vi "Numeric Control - Silver Table.vi"() -> ()   [LabVIEW 2012, in "TableSupportLib.lvlib"]
doc: "Sample numeric display item."
uses:
  TableSupportLib.lvlib
  <vilib>/NI Veristand/Display Template Support/Display Template Support.llb/cluster_Screen Item Settings.ctl
  <vilib>/NI Veristand/Display Template Support/Display Template Support.llb/cluster_Graph Scale Settings.ctl
  <vilib>/NI Veristand/Display Template Support/Display Template Support.llb/cluster_Graph Plot Settings.ctl
  NationalInstruments.VeriStand.SystemStorage
  <vilib>/NI Veristand/Display Template Support/Display Template Support.llb/enum_Display Template Handler Minimal To Widget Msg.ctl
  <vilib>/NI Veristand/Display Template Support/Display Template Support.llb/enum_Display Template Handler Minimal To Workspace.ctl
  SubVIs/Table_StateControl.ctl
  SubVIs/Table_StateInformation.ctl
  SubVIs/Table_ChannelInfoCluster.ctl
  SubVIs/Table_SortArraySettings.ctl
  SubVIs/Table_ListboxSettings.ctl
  <vilib>/NI Veristand/Display Template Support/Display Template Support.llb/sub_Display Template Handler Custom.vi
  <vilib>/NI Veristand/Execution/Workspace/NI VeriStand - Set Single Channel Value.vi
  SubVIs/Table_Globals.vi
  <vilib>/NI Veristand/Execution/Workspace/NI_VS Workspace ExecutionAPI.lvlib
panel:
  in  "Value":dbl
  in  "Listbox":i32(listbox)
  in  "NIVS.Gateway IP Address":string
  in  "NIVS.System Definition Root":refnum<k24>
  in  "Item.Data":T1
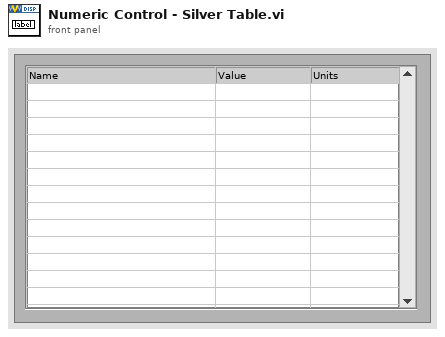
[diagram p1: front panel]
types:
  T1 = typedef "cluster_Screen Item Settings.ctl" = cluster{"Template VI":string, "Position X":i32, "Position Y":i32, "Custom":string, "Show Title Bar":bool, "ID":i32, "Always On Top":bool, "Allow Resize":bool, "Allow Minimize":bool, "Allow Close":bool, "Size to Screen":bool, "Screen.ID":i32, "State":enum16{"Normal", "New"}, "Title":string, "Window Bounds":cluster{"[0]":i16, "[1]":i16, "[2]":i16, "[3]":i16}, "Channel Ref":u64, "Unit":string, "Default Units?":bool, "Flash Limit?":bool, "Color 1":u32, "Color 2":u32, "Color 3":u32, "Color 4":u32, "Bck Color":u32, "Fore Color":u32, "Limit 1":dbl, "Limit 2":dbl, "Limit 3":dbl, "Limit 4":dbl, "Limit Mode 1":i32, "Limit Mode 2":i32, "Limit Mode 3":i32, "Limit Mode 4":i32, "Scale Precision":i32, "Scale Min":dbl, "Scale Max":dbl, "Format":i32, "Precision":i32, "Background Type":i32, "IDs":i32[], "Units":string[], "Labels":string[], "Scale Factor":dbl, "Scale Offset":dbl, "YScale Index":u32[], "XScale":T2, "YScales":T2[], "Plots":T3[], "Update Period":dbl, "History Length":dbl, "My.Ref":refnum<vi>, "Is Control?":bool, "Channel Paths":string[], "Custom Data":variant}
  T2 = typedef "cluster_Graph Scale Settings.ctl" = cluster{"Format":u8, "Precision":u8, "Fit":u8, "Label":string, "Use Default Label":bool, "Label Visible":bool, "Min":dbl, "Max":dbl}
  T3 = typedef "cluster_Graph Plot Settings.ctl" = cluster{"Bar Style":u8, "Fill To":i16, "Fill/PtColor":u32, "Line Style":u8, "Line Width":u8, "Color":u32, "Interp":u8, "Point Style":u8}
  T4 = typedef "TableSupportLib.lvlib/Table_StateControl.ctl" = enum16{"Init", "Run"}
  T5 = typedef "enum_Display Template Handler Minimal To Workspace.ctl" = cluster{"Operation":enum16{"SetCustomData", "DeleteItem"}, "Data":variant}
  T6 = typedef "enum_Display Template Handler Minimal To Widget Msg.ctl" = enum16{"Stop", "LaunchConfigDialog"}
  T7 = typedef "NI_VS Workspace ExecutionAPI.lvlib/WorkspaceAPI.ctl" = refnum<k24>
  T8 = typedef "TableSupportLib.lvlib/Table_StateInformation.ctl" = cluster{"Channel Selection":T9[], "Widths":dbl[], "Sort Info":T10, "Listbox Settings":T11}
  T9 = typedef "TableSupportLib.lvlib/Table_ChannelInfoCluster.ctl" = cluster{"NodePath":string, "Name":string, "Units":string, "Enabled":bool}
  T10 = typedef "TableSupportLib.lvlib/Table_SortArraySettings.ctl" = cluster{"Order":enum16{"ascending", "descending"}, "Column":i32}
  T11 = typedef "TableSupportLib.lvlib/Table_ListboxSettings.ctl" = cluster{"Font":u32, "Bold":bool, "Poll Rate":u32, "Enable Limits":bool, "Path":path}
  T12 = typedef "lveventtype.ctl" = enum32{"Null", "Timeout", "Annotation Menu Selection", "Annotation Menu Selection?", "App Instance Close", "App Instance Close?", "Autoscale Range Change", "Cell Edit", "Cell Edit?", "Cursor Grab", "Cursor Grab?", "Cursor Menu Selection", "Cursor Menu Selection?", "Cursor Move", "Cursor Release", "Data Change", "Direction Change", "Display State Change", "Drag Ended", "Drag Enter", "Drag Leave", "Drag Over", "Drag Source Update", "Drag Starting", "Drag Starting?", "Drop", "Exec State Change", "Key Down", "Key Down?", "Key Repeat", "Key Repeat?", "Key Up", "Listbox Double Click", "Menu Activation?", "Menu Selection (App)", "Menu Selection? (App)", "Menu Selection (User)", "Mouse Down", "Mouse Down?", "Mouse Enter", "Mouse Leave", "Mouse Move", "Mouse Up", "NI Security User Change (App)", "Pane Size", "Panel Close", "Panel Close?", "Panel Resize", "Plot Attribute Change", "Scale Range Change", "Shortcut Menu Activation?", "Shortcut Menu Selection (App)", "Shortcut Menu Selection? (App)", "Shortcut Menu Selection (User)", "Tree Double Click", "Tree Drag", "Tree Drag?", "Tree Drop", "Tree Drop?", "Tree Item Close", "Tree Item Close?", "Tree Item Open", "Tree Item Open?", "Value Change"}
  T13 = typedef "LVPoint32TypeDef.ctl" = cluster{"Horizontal":i32, "Vertical":i32}
  T14 = typedef "LVRowAndColumnTypeDef.ctl" = cluster{"Row":i32, "Column":i32}
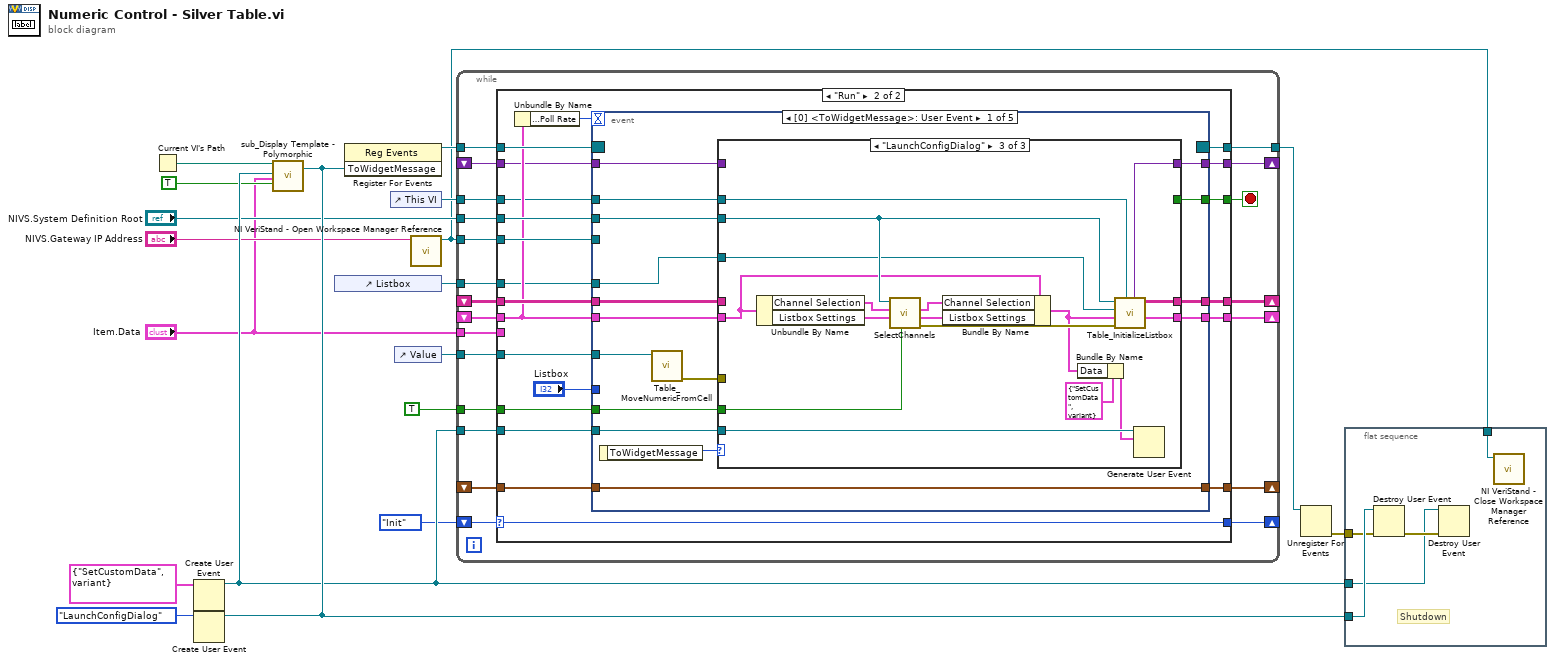
[diagram p0: block diagram]
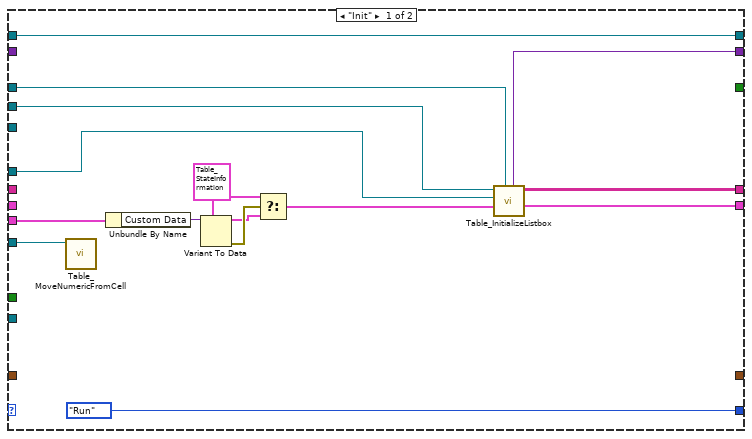
[diagram p2: hidden frame]
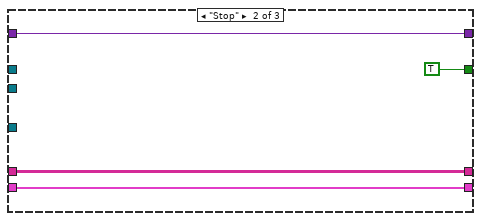
[diagram p4: hidden frame]
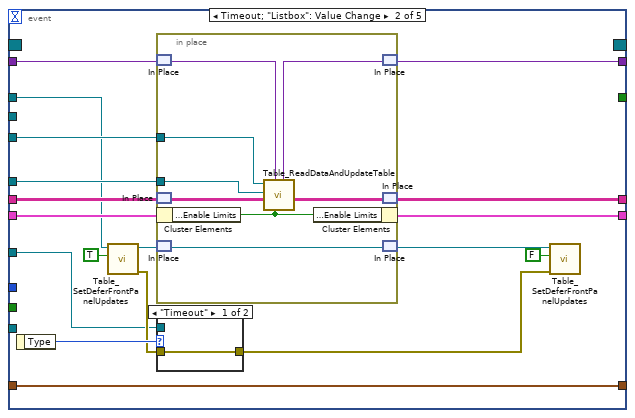
[diagram p5: hidden frame]
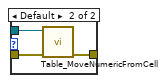
[diagram p6: hidden frame]
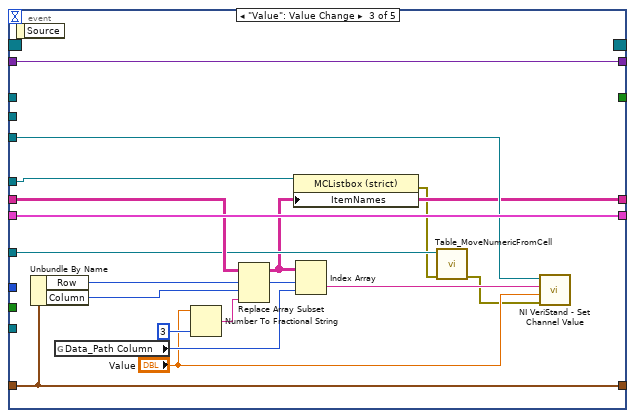
[diagram p7: hidden frame]
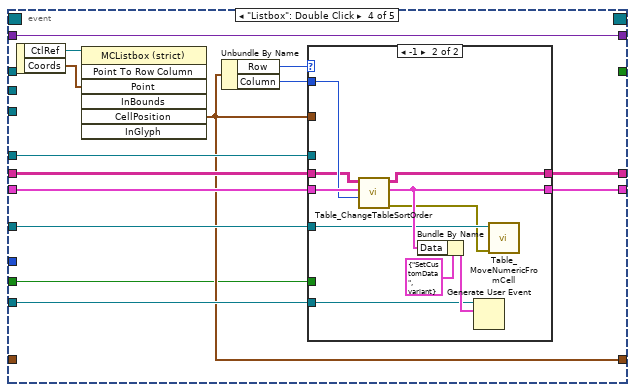
[diagram p8: hidden frame]
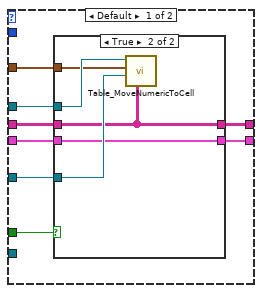
[diagram p9: hidden frame]
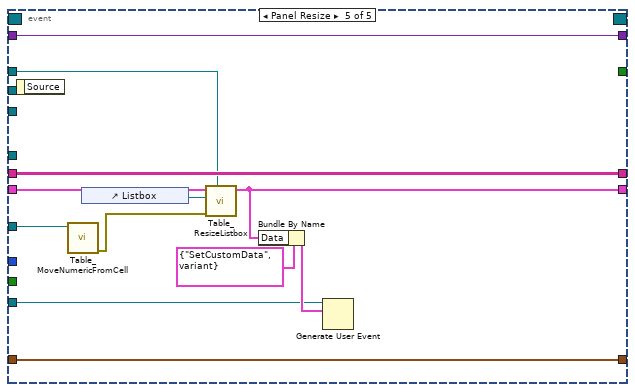
[diagram p11: hidden frame]
diagram:
  n1 = Current VI's Path() -> (path=w12:path)
  n2 = Create User Event(user event datatype=T5 {"Operation"=enum."SetCustomData", "Data"=variant} ("Data")) -> (user event=w11:refnum<user-event>)  [unwired: 1 in, 1 out]
  n3 = Create User Event(user event datatype=enum_Display_Template_Handler_Minimal_To_Widget_Msg."LaunchConfigDialog" ("ToWidgetMessage")) -> (user event=w14:refnum<user-event>)  [unwired: 1 in, 1 out]
  n4 = call-poly <vilib>:"sub_Display Template - Polymorphic.vi"("Parent.Path"=w12, "ToWidgetEvent"=w14, "ToWorkspace"=w11, "Item.Data"="Item.Data", "Resizable"=TRUE) -> ()  [unwired: 1 in, 14 out]
  n5 = control-ref of="Listbox"() -> (w4:refnum<vi>)
  n6 = register-events(w14) -> (reference out=w17:refnum<event-registration>)  [unwired: 2 in, 1 out]
  n7 = control-ref of="This VI"() -> (w5:refnum<vi>)
  n8 = control-ref of="Value"() -> (w3:refnum<vi>)
  n9 = call <vilib>:"NI VeriStand - Open Workspace Manager Reference.vi"("Gateway IP Address (\"\": localhost)"="NIVS.Gateway IP Address") -> ("WorkspaceManager"=w1:T7)  [unwired: 9 in, 1 out]
  n10 = while {
    tunnel: w17 -> [w39]
    tunnel: [w37] -> w16
    tunnel: w11 -> [w36]
    tunnel: "NIVS.System Definition Root" -> [w35]
    shift-right: [w32] -> _
    shift-left: _ -> [w34]
    tunnel: w1 -> [w33]
    shift-right: [w31] -> _
    shift-left: _ -> [w30]
    shift-right: [w28] -> _
    shift-left: Table_StateControl."Init" -> [w29]
    tunnel: "Item.Data" -> [w27]
    shift-right: [w26] -> _
    shift-left: _ -> [w25]
    tunnel: w5 -> [w24]
    tunnel: w4 -> [w23]
    tunnel: w3 -> [w22]
    shift-right: [w21] -> _
    shift-left: _ -> [w20]
    tunnel: TRUE ("Controls Only?") -> [w19]
    stop <- w38 stop-if-true
    n11 = case shown="\"Run\"" w29 {
      selector: w29 -> [_ w66]
      tunnel: w39 -> [w54 w75]
      tunnel: [_ w74] -> w38
      tunnel: [w54 w73] -> w37
      tunnel: w36 -> [_ w72]
      tunnel: w35 -> [w52 w71]
      tunnel: w34 -> [_ w65]
      tunnel: w33 -> [_ w70]
      tunnel: [w51 w69] -> w32
      tunnel: [w50 w68] -> w31
      tunnel: w30 -> [_ w67]
      tunnel: [Table_StateControl."Run" w66] -> w28
      tunnel: w27 -> [w48 _]
      tunnel: [w43 w63] -> w26
      tunnel: w25 -> [_ w62]
      tunnel: w24 -> [w42 w61]
      tunnel: w23 -> [w41 w59]
      tunnel: w22 -> [w40 w58]
      tunnel: [_ w57] -> w21
      tunnel: w20 -> [_ w56]
      tunnel: w19 -> [_ w55]
      frame "Init" {
        w46 = T8 {"Channel Selection"=[], "Widths"=[], "Sort Info"={"Order"=enum."ascending", "Column"=0}, "Listbox Settings"={"Font"=13, "Bold"=FALSE, "Poll Rate"=200, "Enable Limits"=FALSE, "Path"=path ""}}
        n12 = call "Table_MoveNumericFromCell.vi"("Digital in"=w40) -> ()  [unwired: 10 in, 1 out]
        n13 = Unbundle By Name(w48) -> ("Custom Data"=w49:variant)
        n14 = Variant To Data(type=w46, Variant=w49) -> (data=w45:T8, error out=w47:errorcluster)  [unwired: 1 in]
        n15 = Select(t=w46, s=w47, f=w45) -> (s? t:f=w44:T8)
        n16 = call "Table_InitializeListbox.vi"("This VI"=w42, "State Information"=w44, "Listbox Ref"=w41, "NIVS.System Definition Root"=w52) -> ("State Information Out"=w51:T8, "Sorted Array out"=w50:string[][], "Limit Settings"=w43:variant)  [unwired: 3 in, 2 out]
      }
      frame "Run" {
        n17 = Unbundle By Name(w65) -> ("Listbox Settings.Poll Rate"=w64:u32)
        n18 = event shown="[0] <ToWidgetMessage>: User Event" {
          selector: w75 -> [_ _ _ _ _]
          dyn-events: [_ _ _ _ _] -> w73
          timeout: w64 -> [_ _ _ _ _]
          tunnel: [w90 _ _ _ _] -> w74
          tunnel: w72 -> [w89 _ _ w171 w209]
          tunnel: w71 -> [w88 _ _ _ _]
          tunnel: w65 -> [w87 w132 w161 w173 w207]
          tunnel: w70 -> [_ w133 w155 _ _]
          tunnel: [w86 w131 w161 w172 w208] -> w69
          tunnel: [w85 w127 w148 w169 w213] -> w68
          tunnel: w67 -> [w84 w128 w154 w170 w213]
          tunnel: [w83 w129 w162 w168 w206] -> w63
          tunnel: w62 -> [w82 w130 w162 w168 w206]
          tunnel: w61 -> [w81 w124 _ _ w205]
          tunnel: "Listbox" -> [_ _ _ _ _]
          tunnel: w59 -> [w80 w126 w149 w167 _]
          tunnel: w58 -> [w78 w116 w150 w166 w203]
          tunnel: [w79 w120 w160 w165 w204] -> w57
          tunnel: w56 -> [w79 w120 w160 _ w204]
          tunnel: w55 -> [w76 _ _ w163 _]
          event User Event {
            n19 = event-data() -> ("ToWidgetMessage"=w91:T6)  [unwired: 1 out]
            n20 = call "Table_MoveNumericFromCell.vi"("Digital in"=w78) -> ("error out"=w77:errorcluster)  [unwired: 10 in]
            n21 = case shown="\"LaunchConfigDialog\"" w91 {
              tunnel: [_ TRUE _] -> w90
              tunnel: w89 -> [_ _ w115]
              tunnel: w88 -> [_ _ w111]
              tunnel: w87 -> [w94 w97 w109]
              tunnel: [w94 w97 w106] -> w86
              tunnel: [w93 w96 w107] -> w85
              tunnel: w84 -> [w93 w96 _]
              tunnel: [w92 w95 w102] -> w83
              tunnel: w82 -> [w92 w95 _]
              tunnel: w81 -> [_ _ w101]
              tunnel: w80 -> [_ _ w100]
              tunnel: w77 -> [_ _ _]
              tunnel: w76 -> [_ _ w99]
              frame Default {
              }
              frame "Stop" {
              }
              frame "LaunchConfigDialog" {
                n22 = Unbundle By Name(w109) -> ("Channel Selection"=w114:T9[], "Listbox Settings"=w103:T11)
                n23 = call "SelectChannels.vi"("Controls Only?"=w99, "Listbox Settings"=w103, "Previous Selection"=w114, "Root.BaseNodeType"=w111) -> ("error out"=w110:errorcluster, "Listbox Settings Out"=w104:T11, "Channel Selection"=w108:T9[])  [unwired: 5 in]
                n24 = Bundle By Name(cluster=w109, "Channel Selection"=w108, "Listbox Settings"=w104) -> (w105:T8)
                n25 = Bundle By Name(cluster=T5 {"Operation"=enum."SetCustomData", "Data"=variant} ("event data"), "Data"=w105) -> (w112:T5)
                n26 = call "Table_InitializeListbox.vi"("This VI"=w101, "error in (no error)"=w110, "State Information"=w105, "Listbox Ref"=w100, "NIVS.System Definition Root"=w111) -> ("State Information Out"=w106:T8, "Sorted Array out"=w107:string[][], "Limit Settings"=w102:variant)  [unwired: 2 in, 2 out]
                n27 = Generate User Event(user event=w115, event data cluster=w112) -> ()  [unwired: 1 in, 2 out]
              }
            }
          }
          event Timeout; "Listbox": Value Change {
            n28 = event-data() -> ("Type"=w118:T12)  [unwired: 1 out]
            n29 = call "Table_SetDeferFrontPanelUpdates.vi"("Defer Panel Updates"=TRUE, "VI Ref"=w124) -> ("error out"=w117:errorcluster, "VI Ref out"=w123:refnum<vi>)  [unwired: 8 in]
            n30 = in-place {
              in-place-border: w133 -> [w145]
              in-place-border: w126 -> [w139]
              n31 = in-place-match #1(w130) -> (w143:variant)
              n32 = in-place-match #2(w128) -> (w141:string[][])
              n33 = in-place-cluster #3(w132) -> ("Listbox Settings.Enable Limits"=w144:bool)
              n34 = in-place-match #4(w123) -> (w138:refnum<vi>)
              n35 = call "Table_ReadDataAndUpdateTable.vi"("Enable Limits"=w144, "Limit Settings"=w143, "Data"=w141, "Listbox Ref"=w139, "WorkspaceManager"=w145) -> ("Data Out"=w140:string[][], "Limit Settings Out"=w142:variant)  [unwired: 3 in, 2 out]
              n36 = in-place-cluster #3("Listbox Settings.Enable Limits"=w144) -> (w131:T8)
              n37 = in-place-match #1(w142) -> (w129:variant)
              n38 = in-place-match #2(w140) -> (w127:string[][])
              n39 = in-place-match #4(w138) -> (w122:refnum<vi>)
            }
            n40 = case shown="\"Timeout\"" w118 {
              tunnel: [w134 w137] -> w119
              tunnel: w117 -> [w134 w136]
              tunnel: w116 -> [_ w135]
              frame "Timeout" {
              }
              frame Default {
                n41 = call "Table_MoveNumericFromCell.vi"("error in (no error)"=w136, "Digital in"=w135) -> ("error out"=w137:errorcluster)  [unwired: 9 in]
              }
            }
            n42 = call "Table_SetDeferFrontPanelUpdates.vi"("error in (no error)"=w119, "Defer Panel Updates"=FALSE, "VI Ref"=w122) -> ()  [unwired: 7 in, 2 out]
          }
          event "Value": Value Change {
            n43 = event-data() -> ()  [unwired: 2 out]
            n44 = Unbundle By Name(w160) -> ("Row"=w158:i32, "Column"=w159:i32)
            n45 = global read "Table_Globals.vi" "Data_Path Column"() -> (w157:i32)
            n46 = Number To Fractional String(number="Value", precision (6)=i16 3) -> (F-format string=w151:string)  [unwired: 2 in]
            n47 = Replace Array Subset(array=w154, new element=w151, index (row)=w158, index (col)=w159) -> (w148:string[][])
            n48 = property on="Property Node" class="MCListbox (strict)"(reference=w149, "ItemNames"=w148) -> (error out=w147:errorcluster)  [unwired: 1 in, 1 out]
            n49 = Index Array(array=w148, index (row)=w158, index (col)=w157) -> (element=w156:string)
            n50 = call "Table_MoveNumericFromCell.vi"("error in (no error)"=w147, "Digital in"=w150) -> ("error out"=w146:errorcluster)  [unwired: 9 in]
            n51 = call-poly <vilib>:"NI VeriStand - Set Channel Value.vi"("error in (no error)"=w146, "Value"="Value", "Channel"=w156, "WorkspaceManager in"=w155) -> ()  [unwired: 6 in, 2 out]
          }
          event "Listbox": Double Click {
            n52 = event-data() -> ("CtlRef"=w176:refnum<vi>, "Coords"=w175:T13)  [unwired: 1 out]
            n53 = invoke class="MCListbox (strict)" method="Point To Row Column"(reference=w176, "Point"=w175) -> ("CellPosition"=w165:T14)  [unwired: 5 in, 6 out]
            n54 = Unbundle By Name(w165) -> ("Row"=w164:i32, "Column"=w174:i32)
            n55 = case shown="-1" w164 {
              tunnel: w174 -> [_ w195]
              tunnel: w173 -> [w177 w201]
              tunnel: [w178 w197] -> w172
              tunnel: w171 -> [_ w198]
              tunnel: w170 -> [w183 w194]
              tunnel: [w179 w196] -> w169
              tunnel: w167 -> [w184 _]
              tunnel: w165 -> [w182 _]
              tunnel: w166 -> [w181 w193]
              tunnel: w163 -> [w180 _]
              frame Default {
                n56 = case shown="True" w180 {
                  tunnel: w184 -> [_ w191]
                  tunnel: w183 -> [w186 w188]
                  tunnel: w182 -> [_ w190]
                  tunnel: w181 -> [_ w189]
                  tunnel: [w186 w188] -> w179
                  tunnel: [w185 w187] -> w178
                  tunnel: w177 -> [w185 w187]
                  frame False {
                  }
                  frame True {
                    n57 = call "Table_MoveNumericToCell.vi"("Data"=w188, "Numeric"=w189, "Cell Position"=w190, "Listbox"=w191) -> ()  [unwired: 7 in, 1 out]
                  }
                }
              }
              frame -1 {
                n58 = call "Table_ChangeTableSortOrder.vi"("Column"=w195, "State Information in"=w201, "Data In"=w194) -> ("error out"=w192:errorcluster, "State Information out"=w197:T8, "Data Out"=w196:string[][])  [unwired: 6 in]
                n59 = Bundle By Name(cluster=T5 {"Operation"=enum."SetCustomData", "Data"=variant} ("event data"), "Data"=w197) -> (w199:T5)
                n60 = Generate User Event(user event=w198, event data cluster=w199) -> ()  [unwired: 1 in, 2 out]
                n61 = call "Table_MoveNumericFromCell.vi"("error in (no error)"=w192, "Digital in"=w193) -> ()  [unwired: 9 in, 1 out]
              }
            }
          }
          event Panel Resize {
            n62 = event-data() -> ()  [unwired: 2 out]
            n63 = call "Table_MoveNumericFromCell.vi"("Digital in"=w203) -> ("error out"=w202:errorcluster)  [unwired: 10 in]
            n64 = control-ref of="Listbox"() -> (w212:refnum<vi>)
            n65 = call "Table_ResizeListbox.vi"("VI in"=w205, "error in (no error)"=w202, "Listbox Ref"=w212, "State Information"=w207) -> ("State Information Out"=w208:T8)  [unwired: 5 in, 2 out]
            n66 = Bundle By Name(cluster=T5 {"Operation"=enum."SetCustomData", "Data"=variant} ("event data"), "Data"=w208) -> (w210:T5)
            n67 = Generate User Event(user event=w209, event data cluster=w210) -> ()  [unwired: 1 in, 2 out]
          }
        }
      }
    }
  }
  n68 = Unregister For Events(event registration refnum=w16) -> (error out=w15:errorcluster)  [unwired: 1 in]
  n69 = flat-sequence {
    tunnel: w15 -> [w217]
    tunnel: w14 -> [w218]
    tunnel: w11 -> [w215]
    tunnel: w1 -> [w214]
    frame #0 {
      # "Shutdown"
      n70 = Destroy User Event(user event=w218, error in=w217) -> (error out=w216:errorcluster)
      n71 = Destroy User Event(user event=w215, error in=w216) -> ()  [unwired: 1 out]
      n72 = call <vilib>:"NI VeriStand - Close Workspace Manager Reference.vi"("WorkspaceManager"=w214) -> ()  [unwired: 10 in, 1 out]
    }
  }
